vi "Config.vi"(8 "error in (no error)":errorcluster, 11 "MSX-E3701 in":refnum<class "MSX-E3701.lvclass">) -> (0 "error out":errorcluster, 2 "HAL Config Data":T1, 3 "MSX-E3701 out":refnum<class "MSX-E3701.lvclass">)   [LabVIEW 2014, in "MSX-E3701.lvlib" / "MSX-E3701.lvclass"]
doc: "Llama al VI CONFIG PANEL. Saca los datos de Configuración por un cluster."
uses:
  MSX-E3701.lvclass
  DriverMasterSync/build/DriverMasterSync.lvlibp/Modules/HAL/TypeDefs/HAL Config Data.ctl
  DriverMasterSync/build/DriverMasterSync.lvlibp/Modules/HAL/DriverMasterSync/DriverMasterSyncClass/DriverMasterSync.lvclass
  DriverMasterSync/build/DriverMasterSync.lvlibp
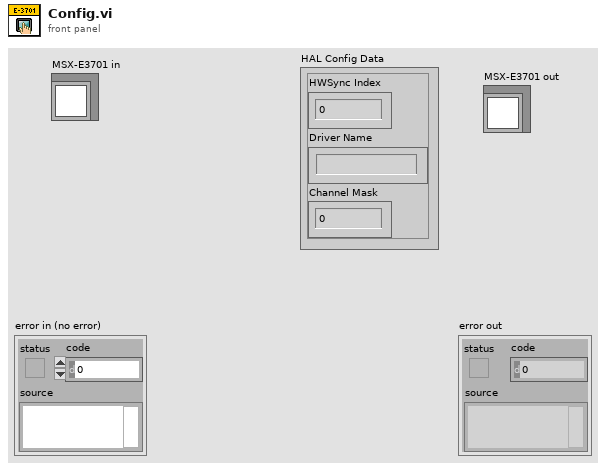
[diagram p1: front panel]
types:
  T1 = typedef "DriverMasterSync.lvlibp/HAL Config Data.ctl" = cluster{"HWSync Index":u32, "Driver Name":string, "Channel Mask":u64}
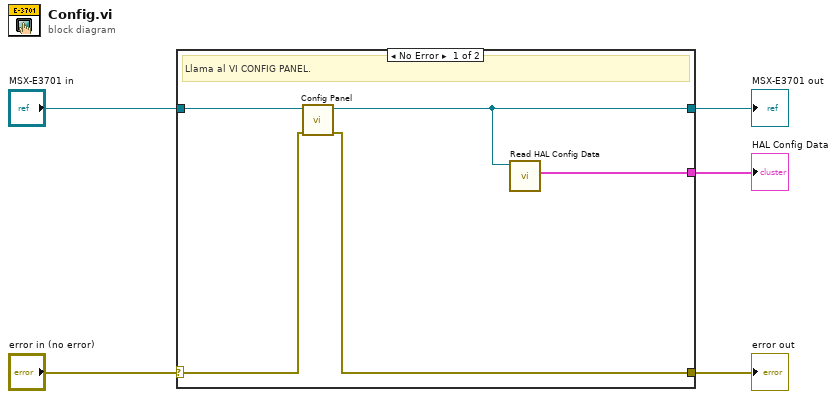
[diagram p0: block diagram]
diagram:
  n1 = case shown="No Error" "error in (no error)" {
    selector: "error in (no error)" -> [w8 w12]
    tunnel: [w7 w12] -> w4
    tunnel: [w10 w11] -> w3
    tunnel: "MSX-E3701 in" -> [w9 w11]
    tunnel: [w6 _] -> w1
    frame No Error {
      # "Llama al VI CONFIG PANEL."
      n2 = call "Config Panel.vi"("Error In"=w8, "MSX-E3701 in"=w9) -> ("Error Out"=w7:errorcluster, "MSX-E3701 out"=w10:refnum<class "MSX-E3701.lvclass">)  [unwired: 7 in]
      n3 = call "Read HAL Config Data.vi"("DriverMasterSync in"=w10) -> ("HAL Config Data"=w6:T1)  [unwired: 8 in, 2 out]
    }
    frame Error {
    }
  }
  "error out" <- w4
  "MSX-E3701 out" <- w3
  "HAL Config Data" <- w1
